vi "Cleanup_IMU_Only.vi"(6 "error in (no error)":errorcluster, 8 "Event Registration Refnum 2":refnum<event-registration>, 9 "IMU Event":refnum<user-event>) -> (3 "Boolean":bool)   [LabVIEW 2014]
uses:
  <userlib>/UCSD Robotics Lab/Robotics-Cape/LV/libroboticscape.lvlib
  Interrupt.lvlib
panel:
  out "function return":i32
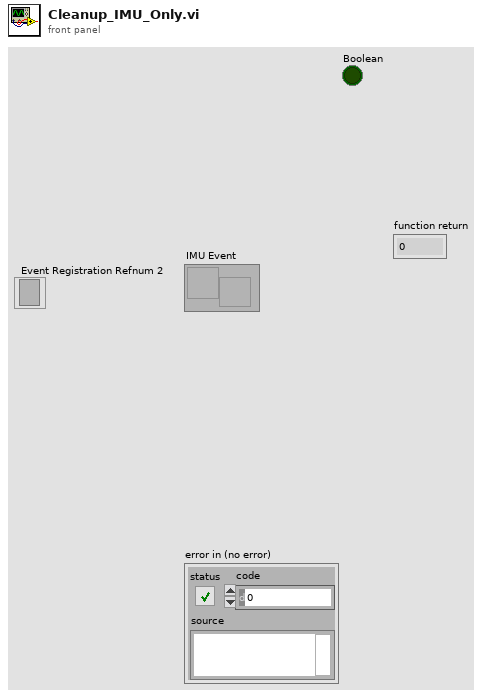
[diagram p1: front panel]
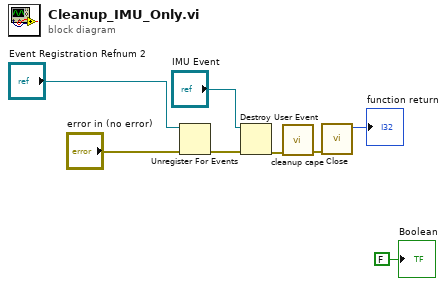
[diagram p0: block diagram]
diagram:
  n1 = Unregister For Events(event registration refnum="Event Registration Refnum 2", error in="error in (no error)") -> (error out=w7:errorcluster)
  n2 = Destroy User Event(user event="IMU Event", error in=w7) -> (error out=w2:errorcluster)
  n3 = call <userlib>:"cleanup cape.vi"("error in (no error)"=w2) -> ("error out"=w3:errorcluster)  [unwired: 9 in, 1 out]
  n4 = call "Close.vi"("error in (no error)"=w3) -> ("function return"=→"function return":i32)  [unwired: 9 in, 1 out]
  "Boolean" <- FALSE ("Boolean")
